vi "ConditionalRefill.vi"(0 "object in":refnum<class "Application.lvclass">, 2 "Turn Off WFG During Refill":bool, 3 "refill below level(uL)":dbl=1000.0, 4 "refill and \nempty rate(uL/min)":dbl=12000.0, 5 "error in (no error)":errorcluster, 9 "Wait After Conditional Refill (s)":dbl=10.0) -> (14 "object out":refnum<class "Application.lvclass">, 19 "error out":errorcluster)   [LabVIEW 2023, in "Application.lvclass"]
uses:
  Application.lvclass
  CetoniPump_class/CetoniPump.lvclass
  InstrumentBase_class/AD2_SDK_class/InstrumentBase.lvclass
  Application.lvclass/Application.ctl
panel:
  in  "Timeout Refill(s)":dbl=80.0 caption="Time Target (s)"
  in  "index":i32
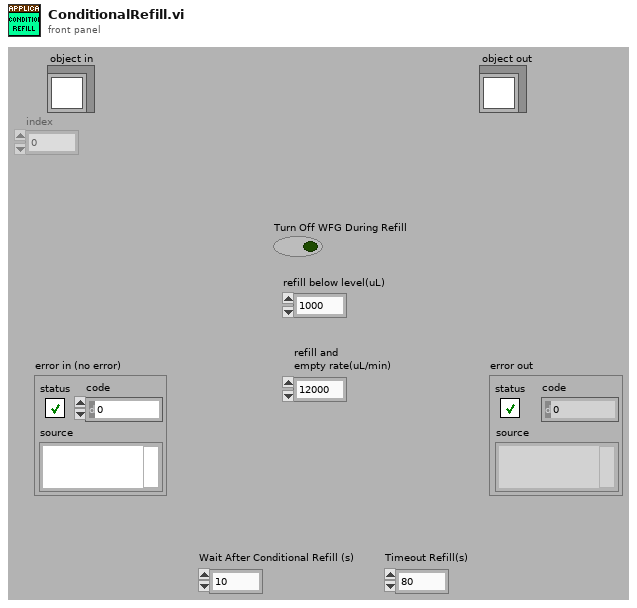
[diagram p1: front panel]
types:
  T1 = cluster{"index":i32, "Level(ml)":dbl, "Flow":dbl}
  T2 = cluster{"Enable Output WFG Ch1":bool, "Enable Output WFG Ch 2":bool}
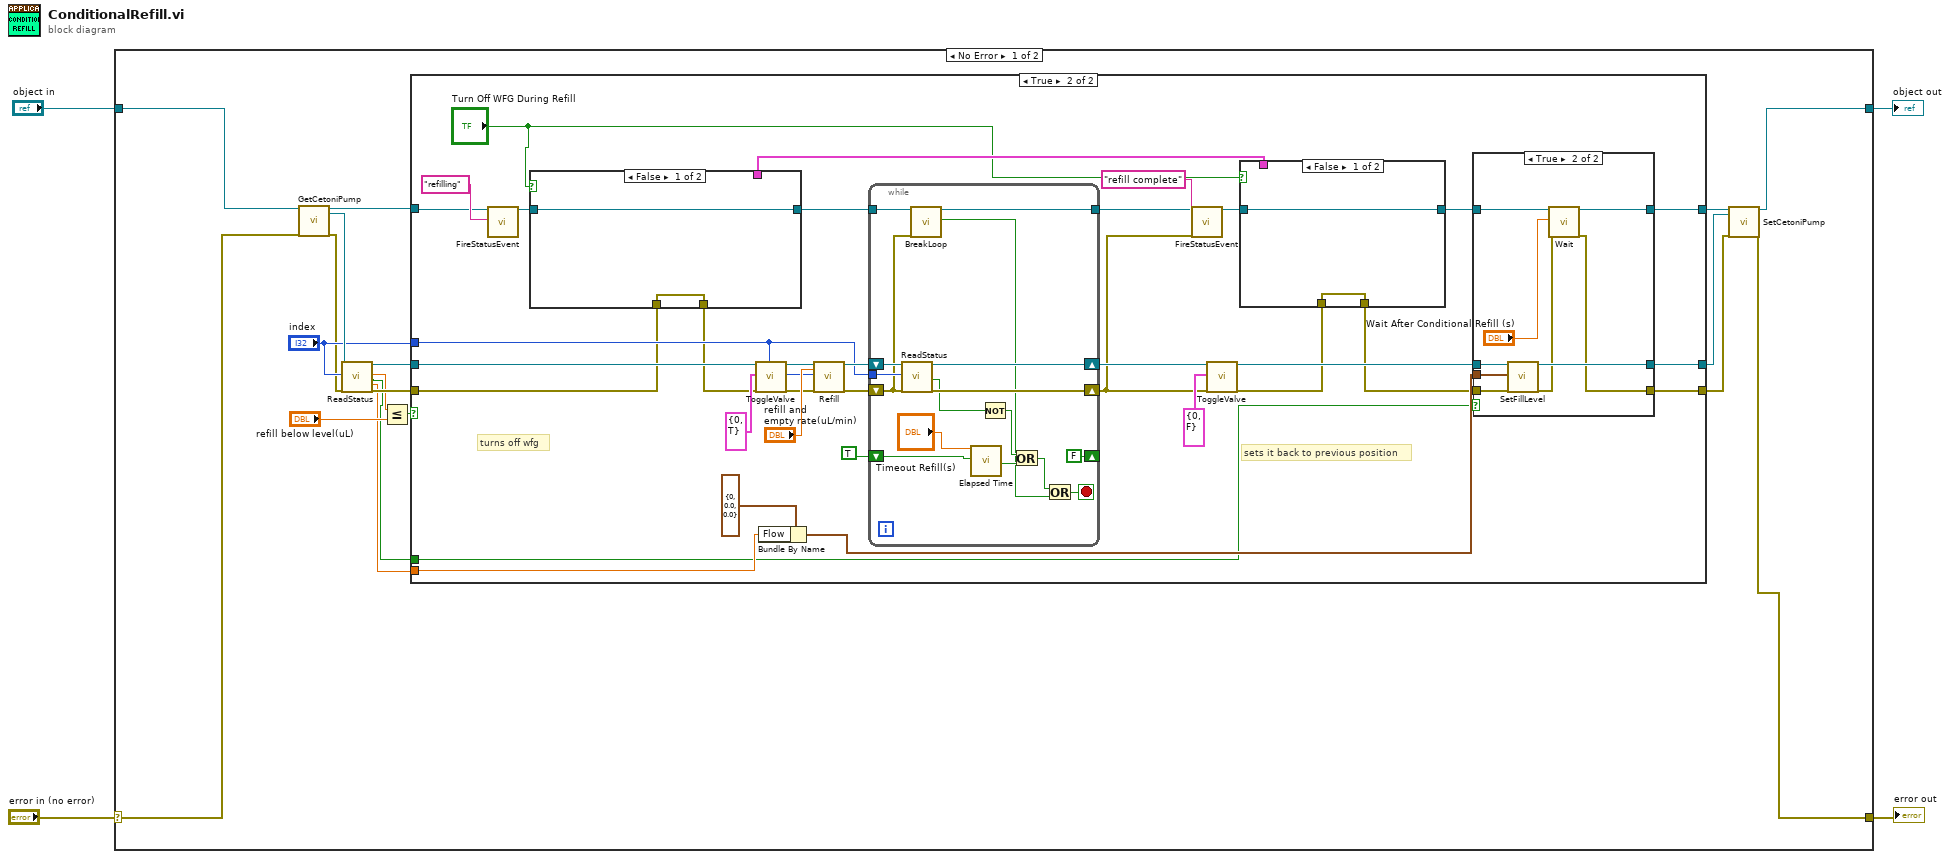
[diagram p0: block diagram]
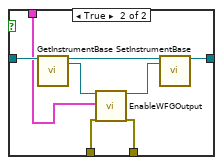
[diagram p3: hidden frame]
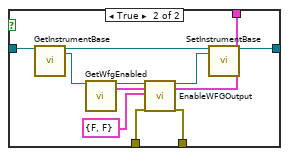
[diagram p4: hidden frame]
diagram:
  n1 = case shown="No Error" "error in (no error)" {
    selector: "error in (no error)" -> [w6 w111]
    tunnel: [w5 w111] -> w3
    tunnel: [w10 w110] -> w1
    tunnel: "object in" -> [w9 w110]
    frame No Error {
      n2 = call-dynamic "GetCetoniPump.vi"("object in"=w9, "error in (no error)"=w6) -> ("object out"=w8:refnum<class "Application.lvclass">, "CetoniPump"=w22:refnum<class "CetoniPump.lvclass">, "error out"=w14:errorcluster)  [unwired: 15 in]
      n3 = call-dynamic "ReadStatus.vi"("object in"=w22, "index"="index", "error in (no error)"=w14) -> ("object out"=w20:refnum<class "CetoniPump.lvclass">, "Fill Level"=w17:dbl, "Is pumping"=w11:bool, "Actual Flow Rate"=w12:dbl, "error out"=w19:errorcluster)  [unwired: 12 in]
      n4 = Less Or Equal?(x=w17, y="refill below level(uL)") -> (x <= y?=w18:bool)
      n5 = case shown="True" w18 {
        tunnel: "index" -> [_ w53]
        tunnel: w20 -> [w25 w51]
        tunnel: w19 -> [w24 w32]
        tunnel: [w25 w44] -> w15
        tunnel: [w24 w43] -> w13
        tunnel: w12 -> [_ w41]
        tunnel: w11 -> [_ w39]
        tunnel: w8 -> [w23 w38]
        tunnel: [w23 w37] -> w7
        frame False {
        }
        frame True {
          # "sets it back to previous position"
          # "turns off wfg"
          n6 = call-dynamic "FireStatusEvent.vi"("object in"=w38, "Status"="refilling") -> ("object out"=w36:refnum<class "Application.lvclass">)  [unwired: 16 in, 1 out]
          n7 = case shown="False" "Turn Off WFG During Refill" {
            tunnel: w36 -> [w71 w81]
            tunnel: [w71 w79] -> w34
            tunnel: [w70 w78] -> w33
            tunnel: w32 -> [w70 w77]
            tunnel: [_ w72] -> w27
            frame False {
            }
            frame True {
              n8 = call-dynamic "GetInstrumentBase.vi"("object in"=w81) -> ("object out"=w80:refnum<class "Application.lvclass">, "InstrumentBase"=w76:refnum<class "InstrumentBase.lvclass">)  [unwired: 16 in, 1 out]
              n9 = call-dynamic "GetWfgEnabled.vi"("object in"=w76) -> ("object out"=w73:refnum<class "InstrumentBase.lvclass">, "WfgEnabled"=w72:cluster{"Ch1":bool, "Ch2":bool})  [unwired: 16 in, 1 out]
              n10 = call-dynamic "EnableWFGOutput.vi"("object in"=w73, "OutputEnable 2"=T2 {"Enable Output WFG Ch1"=FALSE, "Enable Output WFG Ch 2"=FALSE}, "error in (no error)"=w77) -> ("object out"=w75:refnum<class "InstrumentBase.lvclass">, "error out"=w78:errorcluster)  [unwired: 15 in]
              n11 = call-dynamic "SetInstrumentBase.vi"("object in"=w80, "InstrumentBase"=w75) -> ("object out"=w79:refnum<class "Application.lvclass">)  [unwired: 16 in, 1 out]
            }
          }
          n12 = call-dynamic "ToggleValve.vi"("object in"=w51, "ValveControl"=cluster{"index":i32, "Valve Position":bool} {"index"=0, "Valve Position"=TRUE}, "error in (no error)"=w33) -> ("object out"=w52:refnum<class "CetoniPump.lvclass">, "error out"=w50:errorcluster)  [unwired: 15 in]
          n13 = Bundle By Name(cluster=T1 {"index"=0, "Level(ml)"=0.0, "Flow"=0.0} ("GoToLevelSettings"), "Flow"=w41) -> (w40:T1)
          n14 = call-dynamic "Refill.vi"("object in"=w52, "refill rate"="refill and \nempty rate(uL/min)", "index"=w53, "error in (no error)"=w50) -> ("object out"=w59:refnum<class "CetoniPump.lvclass">, "error out"=w58:errorcluster)  [unwired: 14 in]
          n15 = while {
            tunnel: w53 -> [w108]
            shift-right: [w100] -> w48
            shift-left: w59 -> [w109]
            shift-right: [w107] -> w46
            shift-left: w58 -> [w94]
            shift-right: [FALSE] -> _
            shift-left: TRUE -> [w102]
            tunnel: w34 -> [w99]
            tunnel: [w95] -> w35
            stop <- w96 stop-if-true
            n16 = call-dynamic "ReadStatus.vi"("object in"=w109, "index"=w108, "error in (no error)"=w94) -> ("object out"=w100:refnum<class "CetoniPump.lvclass">, "Is pumping"=w105:bool, "error out"=w107:errorcluster)  [unwired: 12 in, 2 out]
            n17 = call-dynamic "BreakLoop.vi"("object in"=w99, "error in (no error)"=w94) -> ("object out"=w95:refnum<class "Application.lvclass">, "Break"=w98:bool)  [unwired: 15 in, 1 out]
            n18 = call "Elapsed Time"("Time Target (s)"="Timeout Refill(s)", "Reset"=w102) -> ("Time has Elapsed"=w103:bool)  [unwired: 10 in, 7 out]
            n19 = Not(x=w105) -> (.not. x?=w104:bool)
            n20 = Or(x=w104, y=w103) -> (x .or. y?=w97:bool)
            n21 = Or(x=w97, y=w98) -> (x .or. y?=w96:bool)
          }
          n22 = call-dynamic "FireStatusEvent.vi"("object in"=w35, "Status"="refill complete", "error in (no error)"=w46) -> ("object out"=w31:refnum<class "Application.lvclass">)  [unwired: 15 in, 1 out]
          n23 = call-dynamic "ToggleValve.vi"("object in"=w48, "ValveControl"=cluster{"index":i32, "Valve Position":bool} {"index"=0, "Valve Position"=FALSE}, "error in (no error)"=w46) -> ("object out"=w45:refnum<class "CetoniPump.lvclass">, "error out"=w29:errorcluster)  [unwired: 15 in]
          n24 = case shown="False" "Turn Off WFG During Refill" {
            tunnel: w31 -> [w61 w66]
            tunnel: [w61 w65] -> w30
            tunnel: w29 -> [w60 w64]
            tunnel: [w60 w63] -> w28
            tunnel: w27 -> [_ w62]
            frame False {
            }
            frame True {
              n25 = call-dynamic "GetInstrumentBase.vi"("object in"=w66) -> ("object out"=w67:refnum<class "Application.lvclass">, "InstrumentBase"=w68:refnum<class "InstrumentBase.lvclass">)  [unwired: 16 in, 1 out]
              n26 = call-dynamic "EnableWFGOutput.vi"("object in"=w68, "OutputEnable 2"=w62, "error in (no error)"=w64) -> ("object out"=w69:refnum<class "InstrumentBase.lvclass">, "error out"=w63:errorcluster)  [unwired: 15 in]
              n27 = call-dynamic "SetInstrumentBase.vi"("object in"=w67, "InstrumentBase"=w69) -> ("object out"=w65:refnum<class "Application.lvclass">)  [unwired: 16 in, 1 out]
            }
          }
          n28 = case shown="True" w39 {
            tunnel: w45 -> [w84 w93]
            tunnel: [w84 w92] -> w44
            tunnel: w28 -> [w83 w91]
            tunnel: [w83 w85] -> w43
            tunnel: w40 -> [_ w90]
            tunnel: w30 -> [w82 w89]
            tunnel: [w82 w87] -> w37
            frame False {
            }
            frame True {
              n29 = call-dynamic "SetFillLevel.vi"("object in"=w93, "GoToLevelSettings"=w90, "error in (no error)"=w91) -> ("object out"=w92:refnum<class "CetoniPump.lvclass">, "error out"=w86:errorcluster)  [unwired: 12 in, 3 out]
              n30 = call-dynamic "Wait.vi"("object in"=w89, "Time Target (s)"="Wait After Conditional Refill (s)", "error in (no error)"=w86) -> ("object out"=w87:refnum<class "Application.lvclass">, "error out"=w85:errorcluster)  [unwired: 15 in]
            }
          }
        }
      }
      n31 = call-dynamic "SetCetoniPump.vi"("object in"=w7, "CetoniPump"=w15, "error in (no error)"=w13) -> ("object out"=w10:refnum<class "Application.lvclass">, "error out"=w5:errorcluster)  [unwired: 15 in]
    }
    frame Error {
    }
  }
  "error out" <- w3
  "object out" <- w1
